vi "Write StepCount.vi"(8 "error in (no error)":errorcluster, 10 "StepCount":u32, 11 "TestDetailedResult in":refnum<class "TestDetailedResult.lvclass">) -> (0 "error out":errorcluster, 3 "TestDetailedResult out":refnum<class "TestDetailedResult.lvclass">)   [LabVIEW 2019, in "TestEngine.lvlib" / "TestDetailedResult.lvclass"]
uses:
  TestDetailedResult.lvclass
  TestDetailedResult.lvclass/TestDetailedResult.ctl
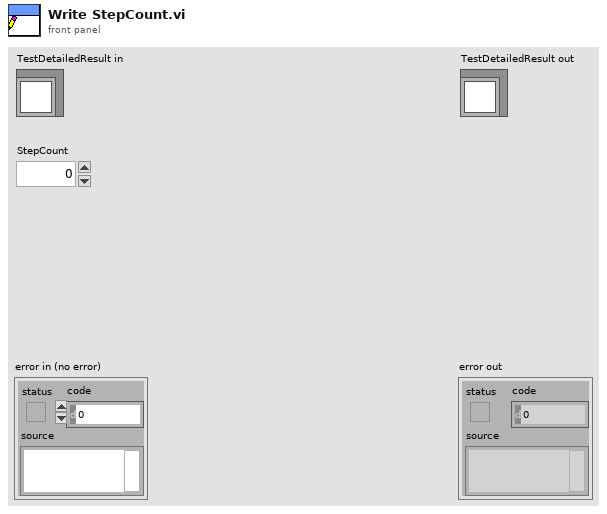
[diagram p1: front panel]
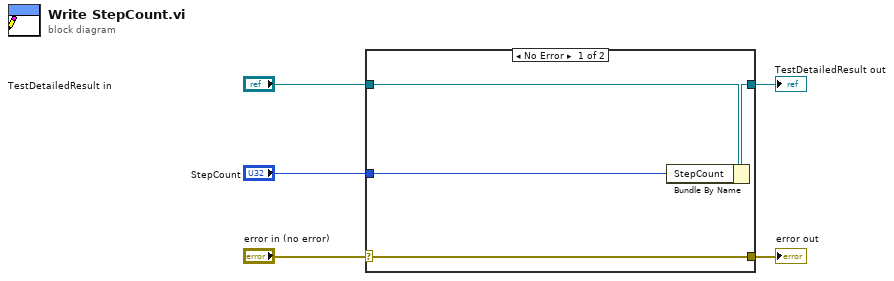
[diagram p0: block diagram]
diagram:
  n1 = case shown="No Error" "error in (no error)" {
    selector: "error in (no error)" -> [w9 w10]
    tunnel: [w9 w10] -> w4
    tunnel: [w7 w11] -> w2
    tunnel: "TestDetailedResult in" -> [w8 w11]
    tunnel: "StepCount" -> [w6 _]
    frame No Error {
      n2 = Bundle By Name(cluster=w8, "StepCount"=w6) -> (w7:refnum<class "TestDetailedResult.lvclass">)
    }
    frame Error {
    }
  }
  "error out" <- w4
  "TestDetailedResult out" <- w2
